vi "ChanotchIndex.vi"(0 "Signal":dbl[](array[numeric]), 1 "Freq":i32[](array[numeric])) -> (2 "Chanotched Signal":dbl[](array[numeric]))   [LabVIEW 2009]
uses:
  <vilib>/Analysis/2dsp.llb/Inverse Complex FFT.vi
  <vilib>/Analysis/2dsp.llb/Real FFT.vi
  <vilib>/Analysis/NI_AALPro.lvlib
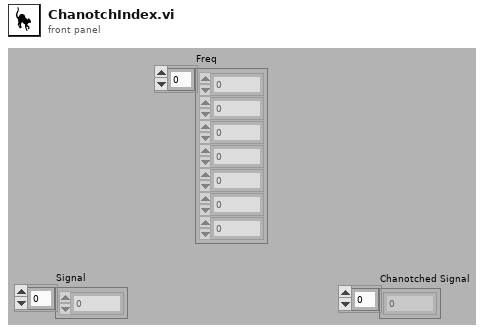
[diagram p1: front panel]
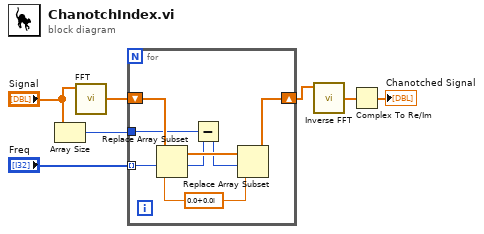
[diagram p0: block diagram]
diagram:
  n1 = Array Size(array="Signal") -> (size(s)=w2:i32)
  n2 = call-poly <vilib>:"FFT.vi"("X"="Signal") -> ("FFT {X}"=w4:cdb[])  [unwired: 9 in, 1 out]
  n3 = for {
    shift-right: [w11] -> w3
    shift-left: w4 -> [w14]
    tunnel: "Freq" -> [w10] mode=indexing
    tunnel: w2 -> [w9]
    w13 = cdb 0.0+0.0i ("nouvel élt/sous-tableau")
    n4 = Replace Array Subset(array=w14, new element=w13, index=w10) -> (w12:cdb[])
    n5 = Subtract(x=w9, y=w10) -> (x-y=w8:i32)
    n6 = Replace Array Subset(array=w12, new element=w13, index=w8) -> (w11:cdb[])
  }
  n7 = call-poly <vilib>:"Inverse FFT.vi"("FFT {X}"=w3) -> ("X"=w6:cdb[])  [unwired: 9 in, 1 out]
  n8 = Complex To Re/Im(x + iy=w6) -> (x=→"Chanotched Signal":dbl[])  [unwired: 1 out]
